vi "New Job Status.vi"(8 "error in (no error)":errorcluster, 9 "Items (unknown)":i32, 10 "Status":string, 11 "Bar in":refnum<class "Bar.lvclass">) -> (0 "error out":errorcluster, 3 "Bar out":refnum<class "Bar.lvclass">)   [LabVIEW 2015, in "Simple Progress Bar.lvlib" / "Bar.lvclass"]
doc: "Display a new <b>Status</b> text in the first progress bar indicator. If greater than zero the <b>Items</b> parameters will size the second progress bar indicator."
uses:
  Class/Bar.lvclass
  Class/Bar.lvclass/Bar.ctl
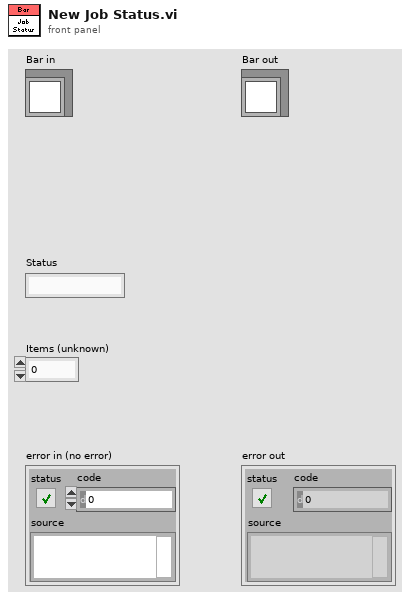
[diagram p1: front panel]
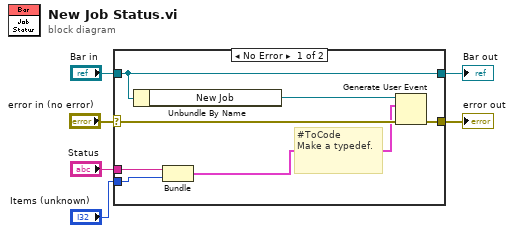
[diagram p0: block diagram]
diagram:
  n1 = case shown="No Error" "error in (no error)" {
    selector: "error in (no error)" -> [w12 w14]
    tunnel: "Bar in" -> [w10 w15]
    tunnel: [w10 w15] -> w1
    tunnel: [w11 w14] -> w5
    tunnel: "Status" -> [w9 _]
    tunnel: "Items (unknown)" -> [w8 _]
    frame No Error {
      # "#ToCode\nMake a typedef."
      n2 = Unbundle By Name(w10) -> ("New Job"=w13:refnum<user-event>)
      n3 = Bundle("Status"=w9, "Items (unknown)"=w8) -> (w7:cluster{"Status":string, "Items (unknown)":i32})  [unwired: 1 in]
      n4 = Generate User Event(user event=w13, event data cluster=w7, error in=w12) -> (error out=w11:errorcluster)  [unwired: 1 in, 1 out]
    }
    frame Error {
    }
  }
  "error out" <- w5
  "Bar out" <- w1
